vi "Get System ID.vi"() -> (3 "SystemID":string)   [LabVIEW 2015, in "SystemLink runtime.lvclass"]
doc: "Returns minion ID of current system or the hostname if the current system does not have a minion ID."
uses:
  SystemLink runtime.lvclass
  <vilib>/Skyline/Utilities/NI Skyline Utilities.lvlib
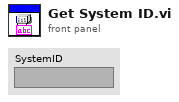
[diagram p1: front panel]
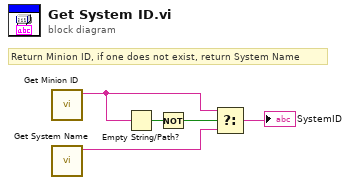
[diagram p0: block diagram]
diagram:
  # "Return Minion ID, if one does not exist, return System Name"
  n1 = call <vilib>:"Get Minion ID.vi"() -> ("minion id"=w3:string)  [unwired: 11 in]
  n2 = call <vilib>:"Get System Name.vi"() -> ("system name"=w4:string)  [unwired: 11 in]
  n3 = Empty String/Path?(string/path=w3) -> (empty?=w1:bool)
  n4 = Not(x=w1) -> (.not. x?=w2:bool)
  n5 = Select(t=w3, s=w2, f=w4) -> (s? t:f=→"SystemID":string)
